vi "Test Chemyx pump control.vi"() -> ()   [LabVIEW 2009]
panel:
  in  "stop":bool
  in  "Stop":bool
  in  "Start":bool
  in  "Update parameters":bool
  out "command string":string
  in  "Syringe Diameter (mm)":dbl=4.61
  in  "withdraw/infuse (1/0)":bool
  in  "Units":dbl=3.0
  in  "Volume (uL)":dbl
  in  "Rate (uL/h)":dbl
  in  "VISA resource name":refnum<visa-resource-name>="COM4"
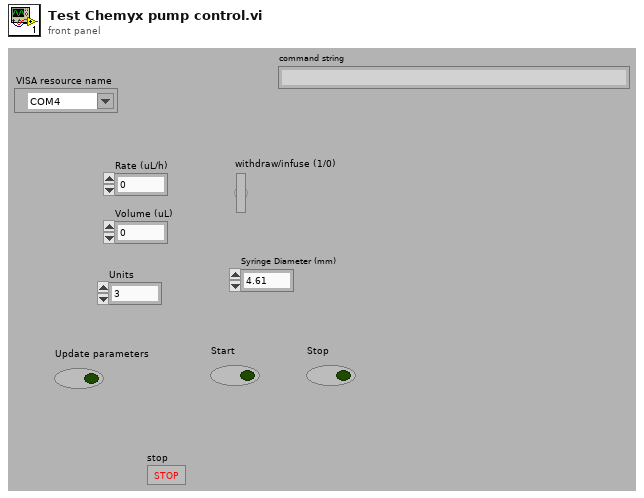
[diagram p1: front panel]
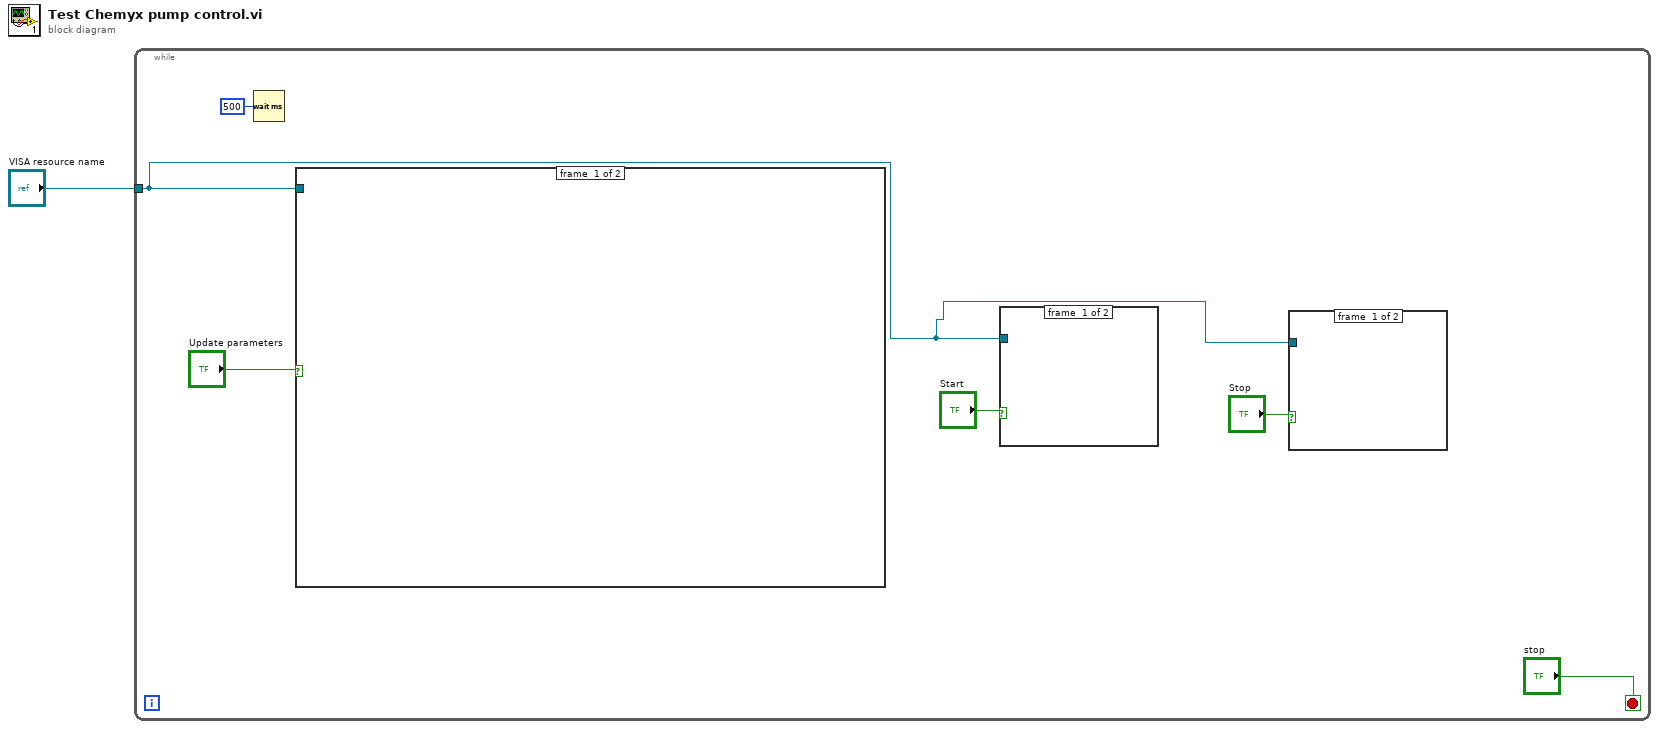
[diagram p0: block diagram]
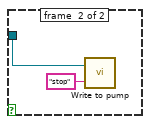
[diagram p2: hidden frame]
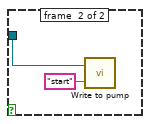
[diagram p3: hidden frame]
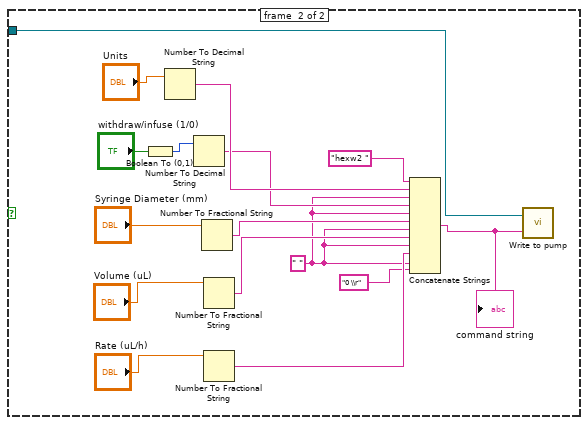
[diagram p4: hidden frame]
diagram:
  n1 = while {
    tunnel: "VISA resource name" -> [w3]
    stop <- "stop" stop-if-true
    n2 = Wait (ms)(milliseconds to wait=u32 500) -> ()  [unwired: 1 out]
    n3 = case shown="True" "Update parameters" {
      tunnel: w3 -> [_ w12]
      frame #0 {
      }
      frame #1 {
        w15 = " " ("string")
        n4 = Boolean To (0,1)(Boolean="withdraw/infuse (1/0)") -> (0, 1=w23:i16)
        n5 = Number To Decimal String(number="Units") -> (decimal integer string=w25:string)  [unwired: 1 in]
        n6 = Number To Decimal String(number=w23) -> (decimal integer string=w22:string)  [unwired: 1 in]
        n7 = Number To Fractional String(number="Syringe Diameter (mm)") -> (F-format string=w20:string)  [unwired: 3 in]
        n8 = Number To Fractional String(number="Volume (uL)") -> (F-format string=w18:string)  [unwired: 3 in]
        n9 = Number To Fractional String(number="Rate (uL/h)") -> (F-format string=w16:string)  [unwired: 3 in]
        n10 = Concatenate Strings("hexw2 " ("string"), w25, w15, w22, w15, w20, w15, w18, w15, w16, w15, "0 \\r" ("string")) -> (w13:string)
        "command string" <- w13
        n11 = call "Write to pump.vi"("string"=w13, "VISA resource name"=w12) -> ()  [unwired: 1 out]
      }
    }
    n12 = case shown="True" "Start" {
      tunnel: w3 -> [_ w11]
      frame #0 {
      }
      frame #1 {
        n13 = call "Write to pump.vi"("string"="start", "VISA resource name"=w11) -> ()  [unwired: 1 out]
      }
    }
    n14 = case shown="True" "Stop" {
      tunnel: w3 -> [_ w9]
      frame #0 {
      }
      frame #1 {
        n15 = call "Write to pump.vi"("string"="stop", "VISA resource name"=w9) -> ()  [unwired: 1 out]
      }
    }
  }
